vi "Cours1.vi"() -> ()   [LabVIEW 2024]
panel:
  out "String 3":string=" Cas vraie"
  in  "stop 2":bool
  in  "Event btn 2":bool
  in  "Event btn":bool
  out "concatenated string":string
  out "String 2":string=" Cas vraie"
  in  "Numeric":u8
  out "substring":string
  out "String":string=" Cas vraie"
  in  "BtnIF":bool
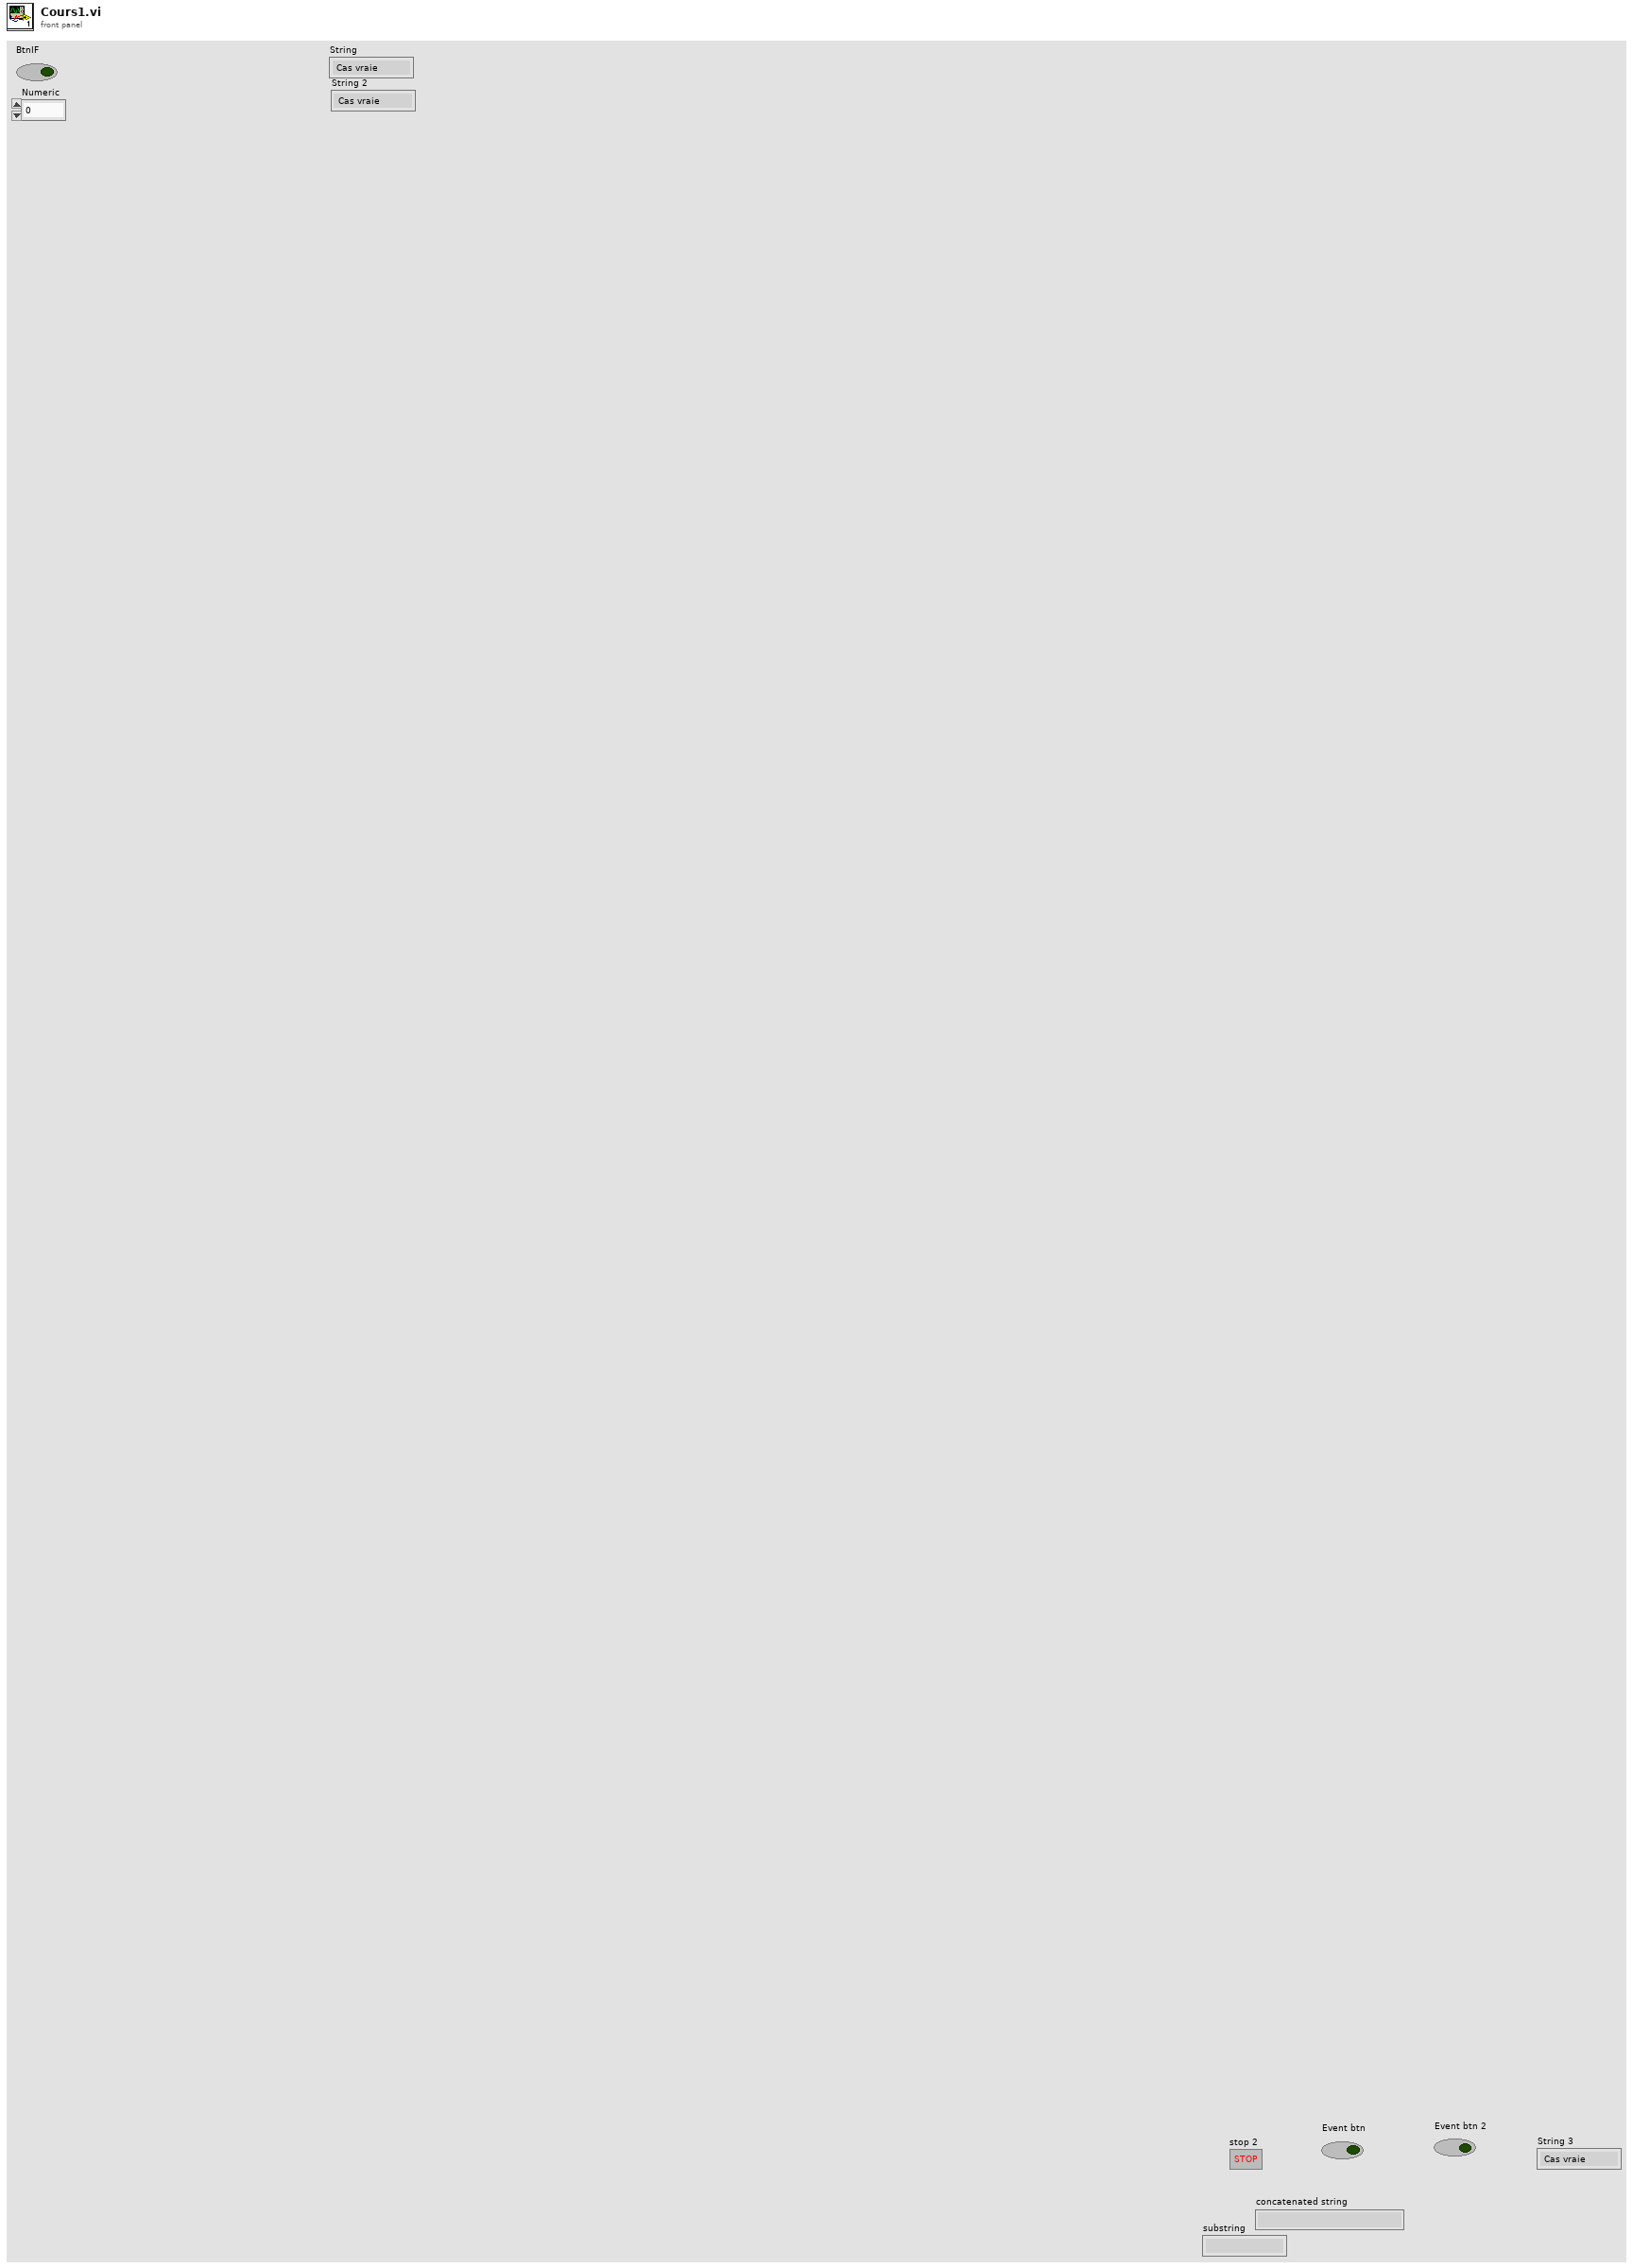
[diagram p1: front panel]
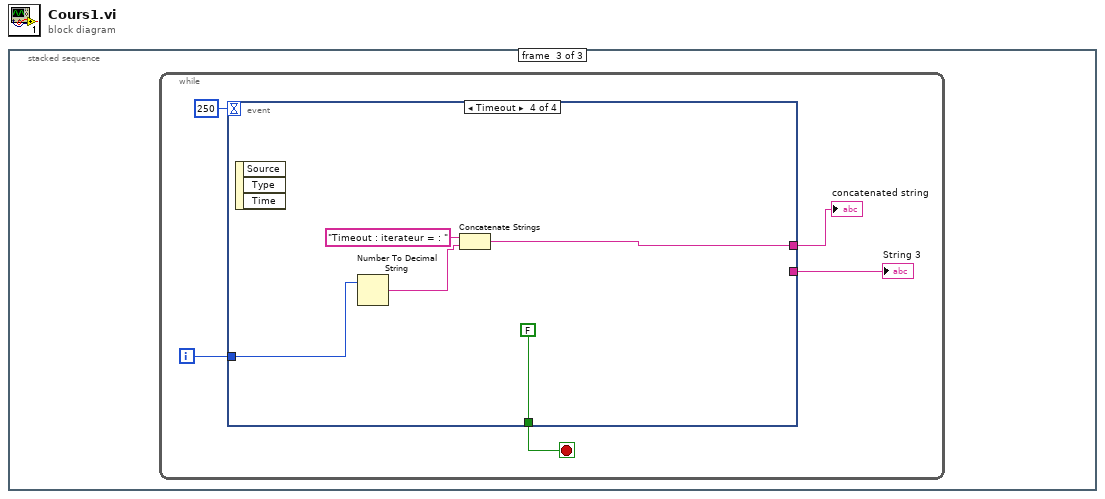
[diagram p0: block diagram]
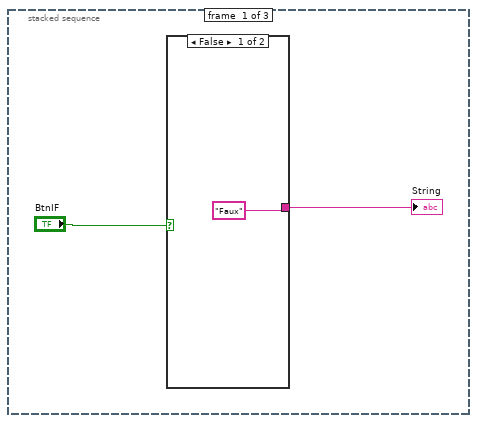
[diagram p2: hidden frame]
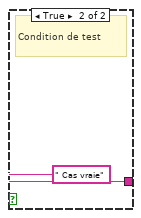
[diagram p3: hidden frame]
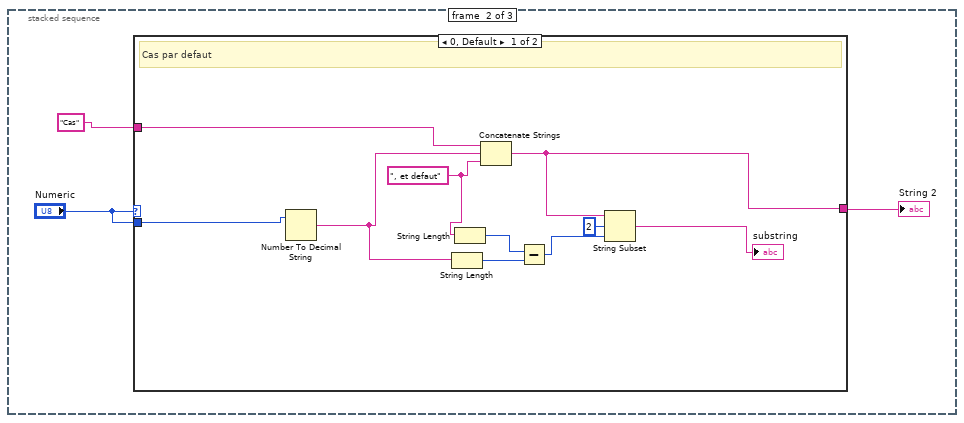
[diagram p4: hidden frame]
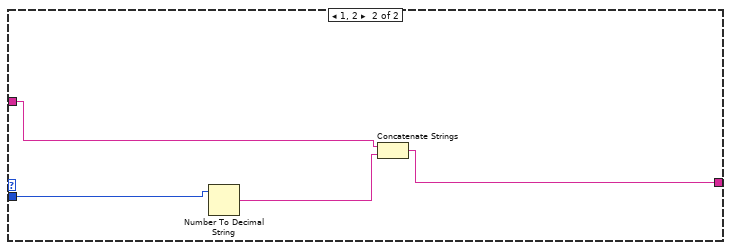
[diagram p5: hidden frame]
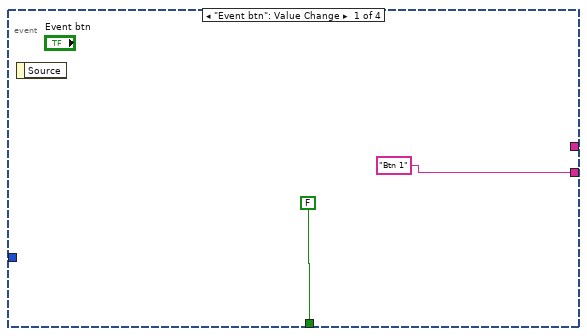
[diagram p6: hidden frame]
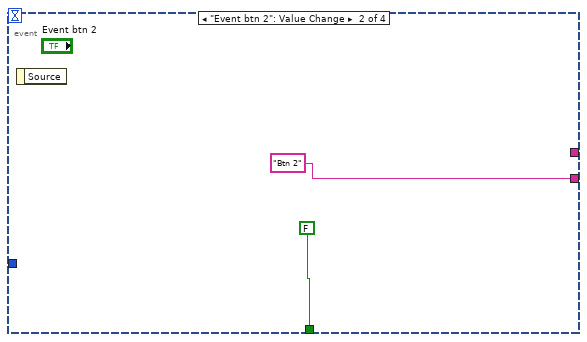
[diagram p7: hidden frame]
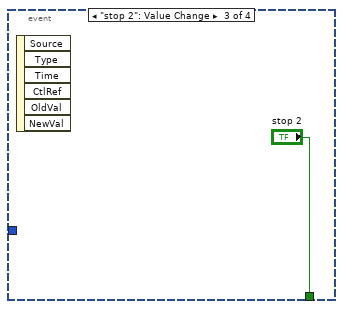
[diagram p8: hidden frame]
diagram:
  n1 = stacked-sequence {
    frame #0 {
      n2 = case shown="False" "BtnIF" {
        tunnel: ["Faux" " Cas vraie"] -> w1
        frame False {
        }
        frame True {
          # "Condition de test"
        }
      }
      "String" <- w1
    }
    frame #1 {
      n3 = case shown="0, Default" "Numeric" {
        tunnel: "Cas" -> [w14 w21]
        tunnel: [w16 w20] -> w6
        tunnel: "Numeric" -> [w17 w19]
        frame 0, Default {
          w8 = ", et defaut" ("string")
          # "Cas par defaut"
          n4 = Number To Decimal String(number=w17) -> (decimal integer string=w12:string)  [unwired: 1 in]
          n5 = String Length(string=w12) -> (length=w11:i32)
          n6 = String Length(string=w8) -> (length=w13:i32)
          n7 = Concatenate Strings(w14, w12, w8) -> (w16:string)
          n8 = Subtract(x=w13, y=w11) -> (x-y=w10:i32)
          n9 = String Subset(string=w16, offset (0)=2, length (rest)=w10) -> (substring=→"substring":string)
        }
        frame 1, 2 {
          n10 = Number To Decimal String(number=w19) -> (decimal integer string=w18:string)  [unwired: 1 in]
          n11 = Concatenate Strings(w21, w18) -> (w20:string)
        }
      }
      "String 2" <- w6
    }
    frame #2 {
      n12 = while {
        i -> [w23]
        stop <- w25 stop-if-true
        n13 = event shown="[3] Timeout" {
          selector: _ -> [_ _ _ _]
          dyn-events: _ -> [_ _ _ _]
          timeout: 250 -> [_ _ _ _]
          tunnel: ["Btn 1" "Btn 2" _ _] -> w26
          tunnel: [FALSE ("stop 2") FALSE ("stop 2") "stop 2" FALSE ("stop 2")] -> w25
          tunnel: w23 -> [_ _ _ w35]
          tunnel: [_ _ _ w32] -> w22
          event "Event btn": Value Change {
            n14 = event-data() -> ()  [unwired: 1 in, 1 out]
          }
          event "Event btn 2": Value Change {
            n15 = event-data() -> ()  [unwired: 1 in, 1 out]
          }
          event "stop 2": Value Change {
            n16 = event-data() -> ()  [unwired: 1 in, 6 out]
          }
          event Timeout {
            n17 = event-data() -> ()  [unwired: 1 in, 3 out]
            n18 = Number To Decimal String(number=w35) -> (decimal integer string=w33:string)  [unwired: 1 in]
            n19 = Concatenate Strings("Timeout : iterateur = : " ("string"), w33) -> (w32:string)
          }
        }
        "String 3" <- w26
        "concatenated string" <- w22
      }
    }
  }
